vi "fsk_test_2.vi"() -> ()   [LabVIEW 2012]
uses:
  <vilib>/addons/Modulation/Digital/General/MT Generate Bits (Galois, PN Order).vi
  <vilib>/addons/Modulation/Digital/General/MT Generate FSK System Parameters(M).vi
  <vilib>/addons/Modulation/niDMT.lvlib
panel:
  out "Waveform Graph 6":dbl[](graph)
  out "Waveform Graph 5":dbl[](graph)
  out "Iterations":i32
  out "Waveform Graph 4":dbl[](graph)
  out "Waveform Graph 3":dbl[](graph)
  out "Waveform Graph 2":dbl[](graph)
  out "Waveform Graph":dbl[](graph)
  out "ber":dbl
  out "error out":errorcluster
  in  "stop":bool
  in  "Total bits":i32=100
  in  "M-FSK":i32=4
  in  "FSK deviation (Hz)":dbl=200000.0
  in  "Symbol rate (Hz)":dbl=1000000.0
  in  "Carrier Frequency (Hz)":dbl=5000000.0
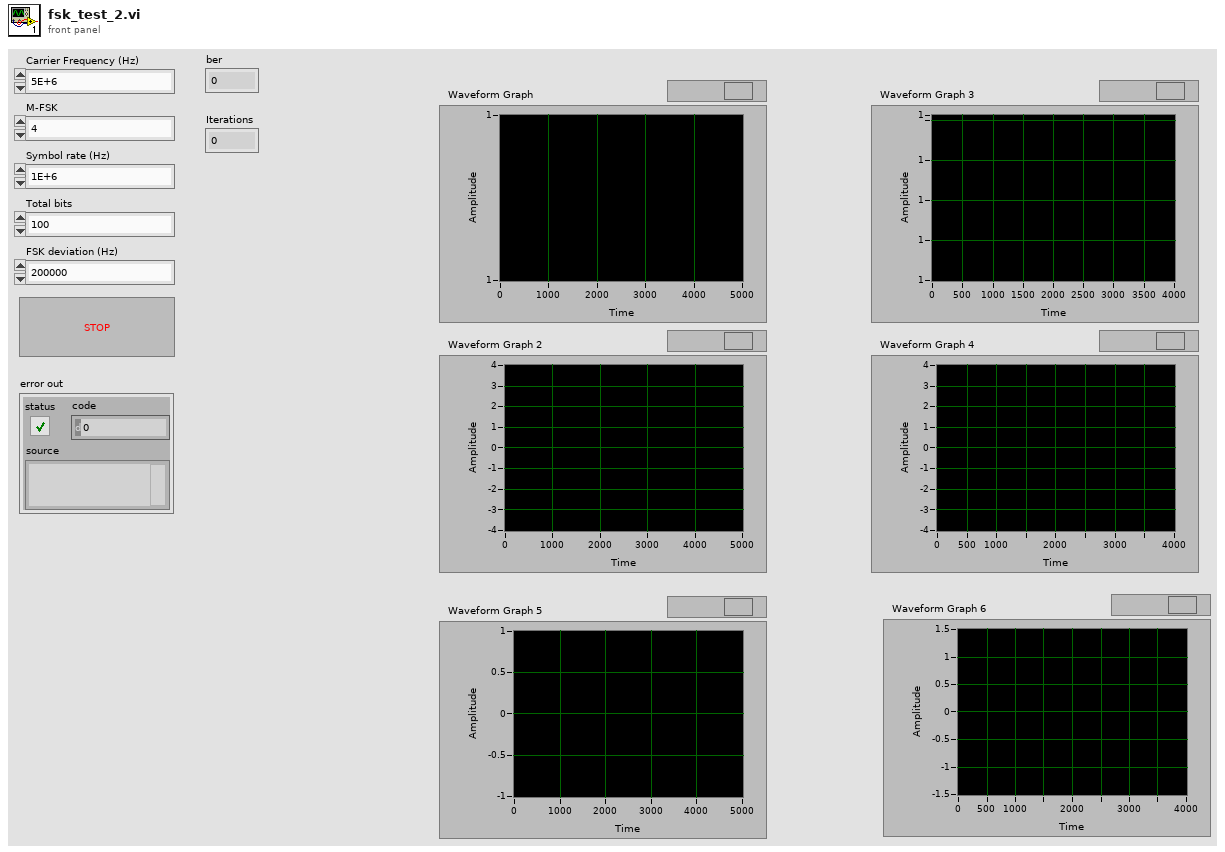
[diagram p1: front panel]
types:
  T1 = cluster{"samples per symbol (16)":i32, "symbol map":dbl[], "symbol phase continuity":enum16{"continuous", "discontinuous"}}
  T2 = typedef "niAMT.lvlib/Complex Data Waveform.ctl" = cluster{"t0":dbl, "dt":dbl, "Y":cdb[]}
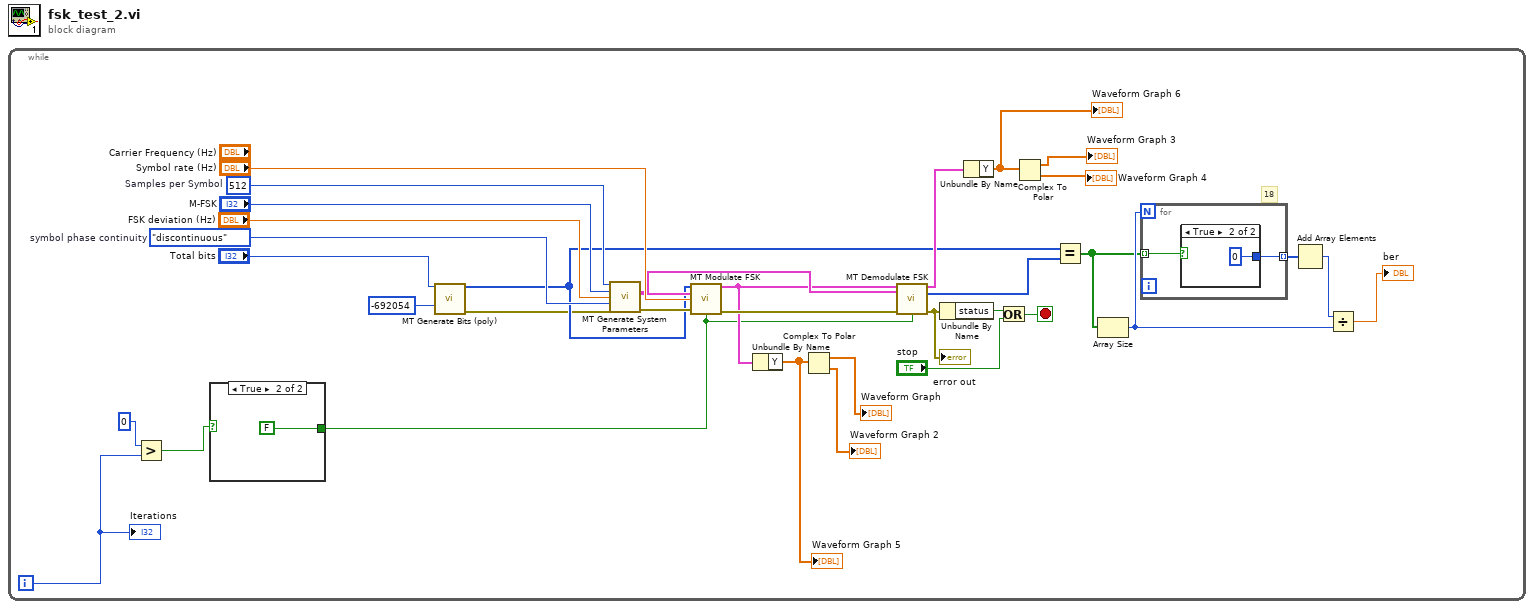
[diagram p0: block diagram]
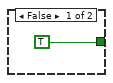
[diagram p2: hidden frame]
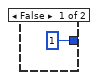
[diagram p3: hidden frame]
diagram:
  n1 = while {
    i -> [w8]
    stop <- w33 stop-if-true
    w30 = enum16{"continuous", "discontinuous"}."discontinuous"  # symbol phase continuity
    w32 = 512  # Samples per Symbol
    # "18"
    n2 = Greater?(x=0, y=w8) -> (0:w9:bool)
    n3 = case shown="True" w9 {
      tunnel: [TRUE FALSE] -> w7
      frame False {
      }
      frame True {
      }
    }
    n4 = call-poly <vilib>:"MT Generate Bits (poly).vi"("total bits (128)"="Total bits", "seed in (0xD6BF7DF2)"=-692054) -> ("output bit stream"=w4:i8[], "error out"=w3:errorcluster)  [unwired: 11 in, 1 out]
    n5 = call-poly <vilib>:"MT Generate System Parameters.vi"("samples per symbol (16)"=w32, "M-FSK (2)"="M-FSK", "FSK deviation (Hz)"="FSK deviation (Hz)", "symbol phase continuity"=w30, "error in (no error)"=w3) -> ("FSK system parameters"=w24:T1, "error out"=w29:errorcluster)  [unwired: 8 in, 1 out]
    n6 = call <vilib>:"MT Modulate FSK.vi"("input bit stream"=w4, "FSK system parameters"=w24, "symbol rate (Hz)"="Symbol rate (Hz)", "error in (no error)"=w29, "reset? (T)"=w7) -> ("output complex waveform"=w16:T2, "error out"=w25:errorcluster)  [unwired: 8 in, 1 out]
    n7 = Unbundle By Name(w16) -> ("Y"=w6:cdb[])
    "Waveform Graph 5" <- w6
    n8 = Complex To Polar(r * e^(i*theta)=w6) -> (r=→"Waveform Graph":dbl[], theta=→"Waveform Graph 2":dbl[])
    n9 = call <vilib>:"MT Demodulate FSK.vi"("input complex waveform"=w16, "FSK system parameters"=w24, "error in (no error)"=w25, "reset? (T)"=w7) -> ("recovered complex waveform"=w15:T2, "output bit stream"=w17:i8[], "error out"=w23:errorcluster)  [unwired: 7 in, 2 out]
    "error out" <- w23
    n10 = Unbundle By Name(w23) -> ("status"=w26:bool)
    n11 = Unbundle By Name(w15) -> ("Y"=w5:cdb[])
    "Waveform Graph 6" <- w5
    n12 = Or(x=w26, y="stop") -> (x .or. y?=w33:bool)
    n13 = Complex To Polar(r * e^(i*theta)=w5) -> (r=→"Waveform Graph 3":dbl[], theta=→"Waveform Graph 4":dbl[])
    n14 = Equal?(x=w4, y=w17) -> (x = y?=w19:bool[])
    n15 = Array Size(array=w19) -> (size(s)=w20:i32)
    n16 = for {
      N: w20 -> [_]
      tunnel: [w38] -> w22 mode=indexing
      tunnel: w19 -> [w37] mode=indexing
      n17 = case shown="True" w37 {
        tunnel: [1 0] -> w38
        frame False {
        }
        frame True {
        }
      }
    }
    n18 = Add Array Elements(numeric array=w22) -> (sum=w21:i32)
    n19 = Divide(x=w21, y=w20) -> (x/y=→"ber":dbl)
    "Iterations" <- w8
  }
